vi "Global Flir-Ax8.vi"() -> ()   [LabVIEW 2016]
panel:
  in  "Image & Doc":path
  in  "Temperature Vector":dbl[](array[numeric])
  in  "Closest Color":u32
  out "Palette":u32[][](array[numeric])
  out "Stop All Loops":bool
  out "M-B Confirm":bool
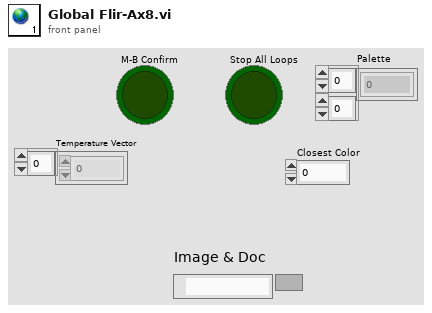
[diagram p1: front panel]
diagram:
